vi "Get Tree Data.vi"(8 "error in":errorcluster, 11 "Tree ref":refnum<vi>) -> (0 "error out":errorcluster, 3 "Array":string[][](array[string]))   [LabVIEW 2025, in "CAN-LIN Raw Bus Capture UI.lvlib"]
uses:
  CAN-LIN Raw Bus Capture UI.lvlib
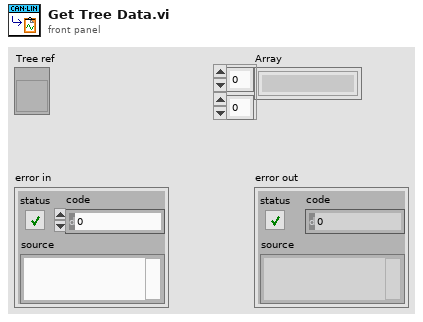
[diagram p1: front panel]
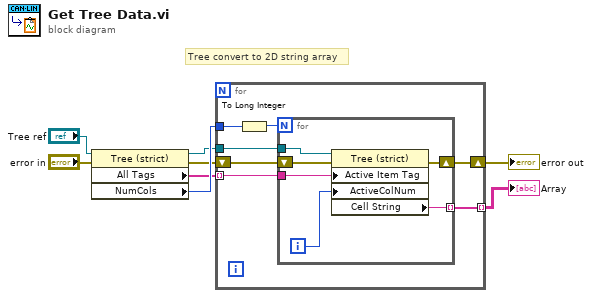
[diagram p0: block diagram]
diagram:
  # "Tree convert to 2D string array"
  n1 = property class="Tree (strict)"(reference="Tree ref", error in="error in") -> (reference out=w3:refnum<vi>, error out=w5:errorcluster, "All Tags"=w7:string[], "NumCols"=w8:u32)
  n2 = for {
    tunnel: w3 -> [w15]
    tunnel: w7 -> [w14] mode=indexing
    tunnel: w8 -> [w11]
    tunnel: [w13] -> w2 mode=indexing
    shift-right: [w9] -> w4
    shift-left: w5 -> [w10]
    n3 = To Long Integer(number=w11) -> (32bit integer=w12:i32)
    n4 = for {
      N: w12 -> [_]
      tunnel: w15 -> [w21]
      tunnel: w14 -> [w20]
      tunnel: [w18] -> w13 mode=indexing
      shift-right: [w16] -> w9
      shift-left: w10 -> [w17]
      i -> [w19]
      n5 = property class="Tree (strict)"(reference=w21, error in=w17, "Active Item Tag"=w20, "ActiveColNum"=w19) -> (error out=w16:errorcluster, "Cell String"=w18:string)  [unwired: 1 out]
    }
  }
  "Array" <- w2
  "error out" <- w4
